vi "enter athlete.vi"() -> ()   [LabVIEW 2009]
uses:
  <vilib>/Utility/file.llb/Write To Spreadsheet File (string).vi
  <vilib>/Utility/file.llb/Read From Spreadsheet File (DBL).vi
panel:
  in  "Data file":path caption="DATA FILE"
  in  "Athlete name":string
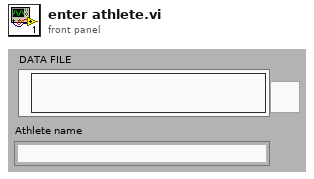
[diagram p1: front panel]
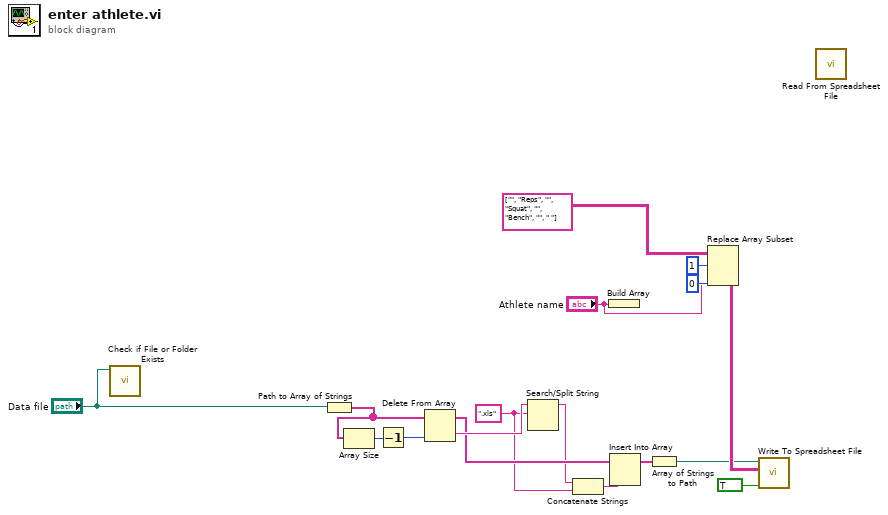
[diagram p0: block diagram]
diagram:
  w3 = ".xls" ("regular expression (\"\")")
  n1 = call <vilib>:"Check if File or Folder Exists.vi"("path"="Data file") -> ()  [unwired: 8 in, 3 out]
  n2 = Path to Array of Strings(0:"Data file") -> (2:w14:string[])  [unwired: 1 out]
  n3 = Array Size(array=w14) -> (size(s)=w13:i32)
  n4 = Decrement(x=w13) -> (x-1=w12:i32)
  n5 = Delete From Array(array=w14, index=w12) -> (deleted portion=w11:string, array with subset deleted=w10:string[])  [unwired: 1 in]
  n6 = Search/Split String(string=w11, search string/char (-)=w3) -> (substring before match=w4:string)  [unwired: 1 in, 2 out]
  n7 = Concatenate Strings(w4, w3) -> (w2:string)
  n8 = Build Array("Athlete name") -> ()  [unwired: 1 out]
  n9 = Insert Into Array(array=w10, new element=w2) -> (w9:string[])  [unwired: 1 in]
  n10 = Array of Strings to Path(0:w9) -> (2:w15:path)  [unwired: 1 in]
  n11 = Replace Array Subset(array=string[][] [["", "Reps"], ["", "Squat"], ["", "Bench"], ["", " "]], new element="Athlete name", index (row)=1, index (col)=0 ("disabled index (col)")) -> (w16:string[][])
  n12 = call-poly <vilib>:"Write To Spreadsheet File.vi"("append to file? (new file:F)"=TRUE, "2D data"=w16, "file path (dialog if empty)"=w15) -> ()  [unwired: 5 in, 1 out]
  n13 = call-poly <vilib>:"Read From Spreadsheet File.vi"() -> ()  [unwired: 7 in, 5 out]
